vi "Basic Output demo.vi"() -> ()   [LabVIEW 2013]
panel:
  out "x .or. y?":bool
  in  "keyboard loop (ms)":u32=150
  in  "mouse loop (ms)":u32=100
  in  "keyboard service name":string="keyboard"
  in  "mouse service name":string="mouse"
  in  "Server address":string
  in  "trig left down":bool
  in  "trig left up":bool=TRUE
  in  "mode":T1(ring)
  out "Mouse Co-ords":T2
  in  "stop":bool
  out "Output (VKeys)":u8[](array[ring])
  # "Paste server address here!"
  # "SERVER DETAILS"
  # "TCP IP FOR KEYBOARD"
  # "&"
  # "DATASOCKET DETAILS  FOR MOUSE"
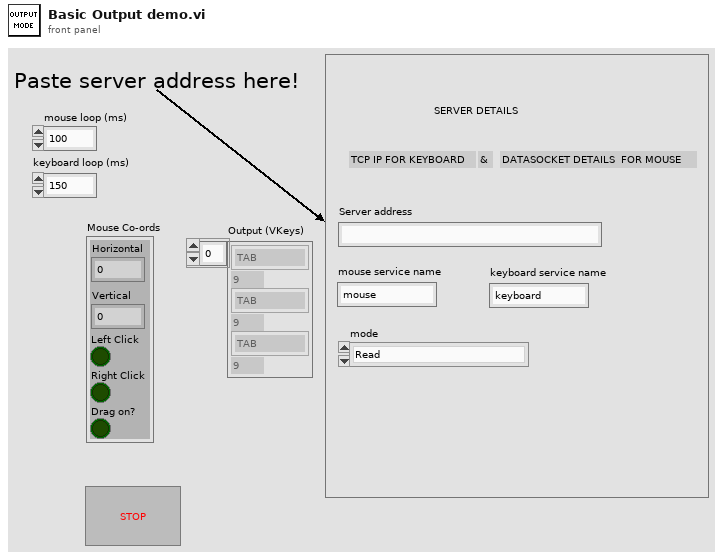
[diagram p1: front panel]
types:
  T1 = enum16{"Read", "Write", "ReadWrite", "BufferedRead", "BufferedReadWrite"}
  T2 = cluster{"Horizontal":i32, "Vertical":i32, "Left Click":bool, "Right Click":bool, "Drag on?":bool}
  T3 = enum16{"0", "1", "2", "3", "4", "5", "6", "7", "8", "9", "A", "B", "C", "D", "E", "F", "G", "H", "I", "J", "K", "L", "M", "N", "O", "P", "Q", "R", "S", "T", "U", "V", "W", "X", "Y", "Z", "F1", "F2", "F3", "F4", "F5", "F6", "F7", "F8", "F9", "F10", "F11", "F12", "F13", "F14", "F15", "ADD", "BACK", "BACKSLASH", "CAPITAL", "COMMA", "DECIMAL", "DELETE", "DIVIDE", "DOWN", "END", "EQUALS", "ESCAPE", "GRAVE (`)", "HOME", "INSERT", "LBRACKET", "LCONTROL", "LEFT", "L ALT", "LSHIFT", "LWIN", "MINUS", "MULTIPLY", "NEXT", "NUMLOCK", "NUMPAD_0", "NUMPAD_1", "NUMPAD_2", "NUMPAD_3", "NUMPAD_4", "NUMPAD_5", "NUMPAD_6", "NUMPAD_7", "NUMPAD_8", "NUMPAD_9", "PAUSE", "PERIOD", "PRIOR (PG UP)", "RBRACKET", "RCONTROL", "RETURN", "RIGHT", "R ALT", "RSHIFT", "RWIN", "SCROLL", "SEMICOLON", "SLASH", "SPACE", "SUBTRACT", "TAB", "UP", "ENTER (num pad)", "' (quote)"}[]
  T4 = cluster{" Key":u8, "Action":enum16{"Press", "Up", "Down"}, "Delay (ms)":u32}
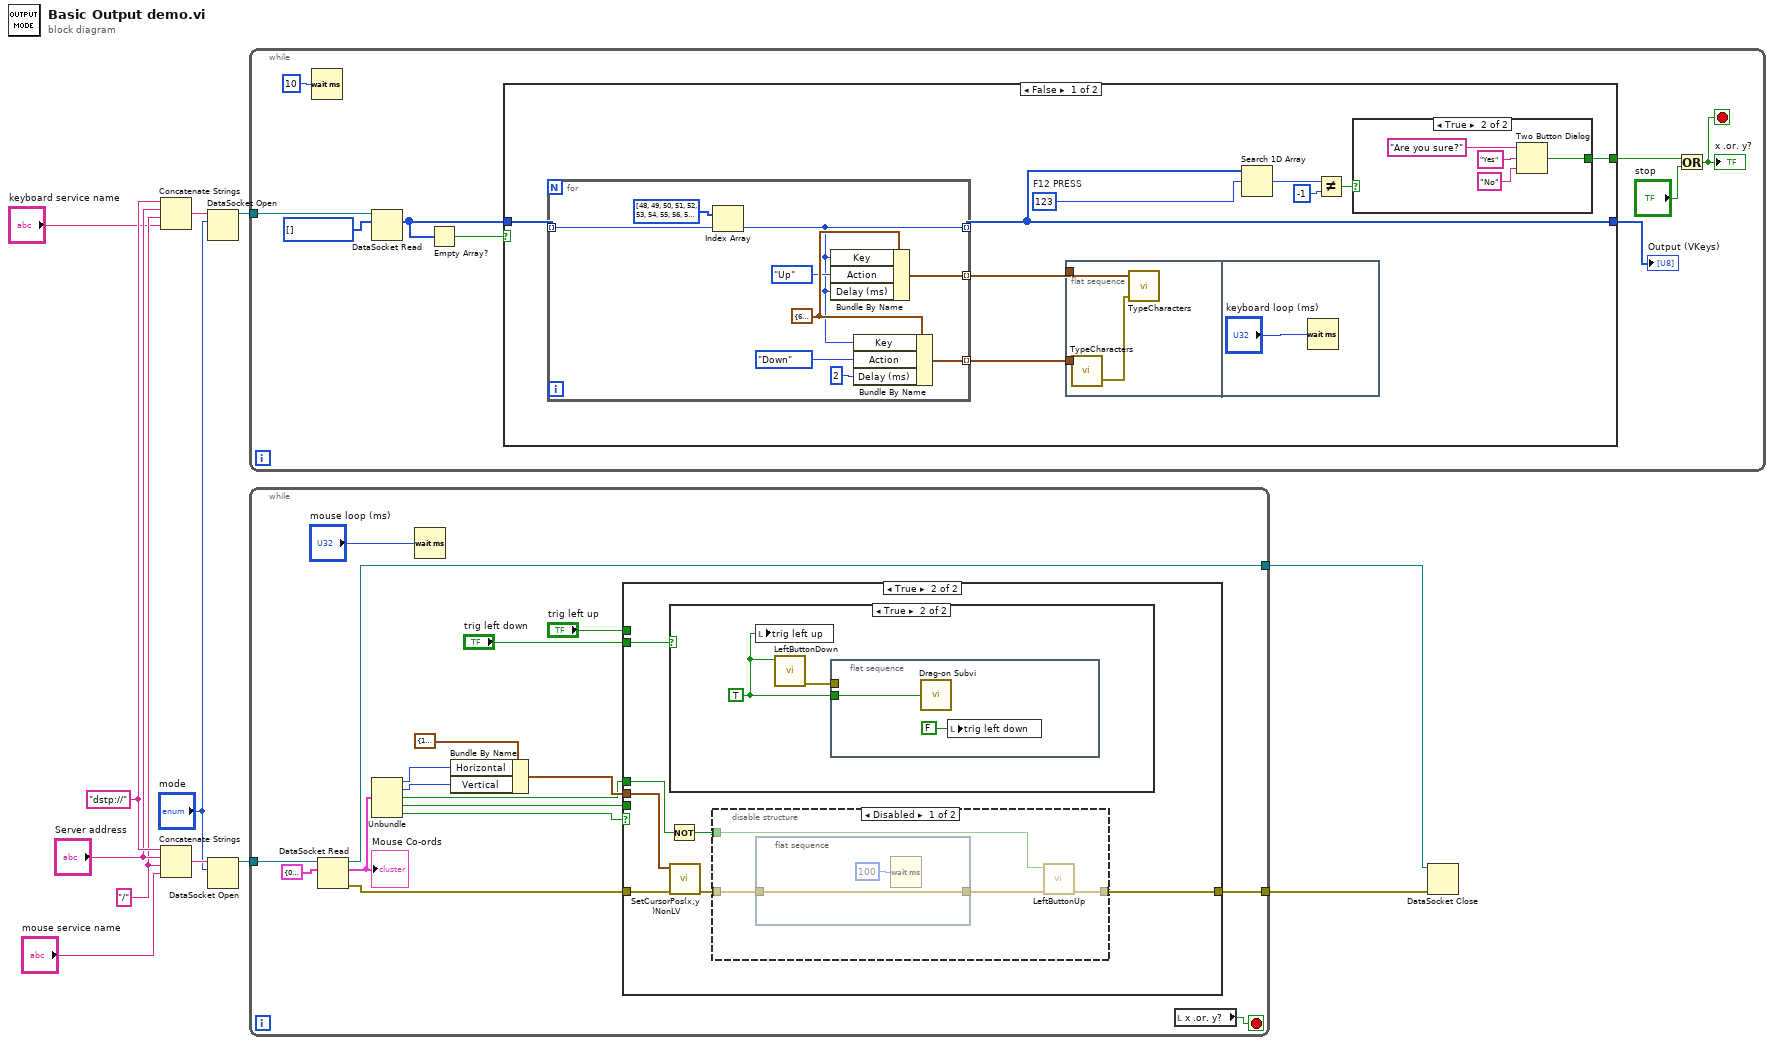
[diagram p0: block diagram]
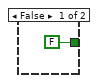
[diagram p2: hidden frame]
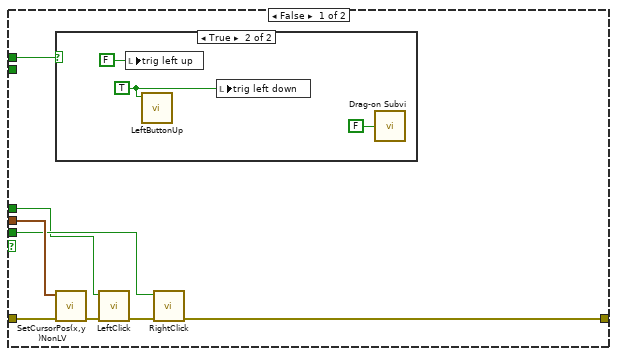
[diagram p4: hidden frame]
diagram:
  w5 = "/" ("string")
  w7 = "dstp://" ("string")
  n1 = Concatenate Strings(w7, "Server address", w5, "keyboard service name") -> (w3:string)
  n2 = Concatenate Strings(w7, "Server address", w5, "mouse service name") -> (w8:string)
  n3 = DataSocket Open(10:"mode", 11:w3) -> (3:w1:refnum<k13>)  [unwired: 2 in, 1 out]
  n4 = DataSocket Open(10:"mode", 11:w8) -> (3:w12:refnum<k13>)  [unwired: 2 in, 1 out]
  n5 = while {
    tunnel: w1 -> [w19]
    stop <- w20 stop-if-true
    w18 = T3 [] items=["0", "1", "2", "3", "4", "5", "6", "7", "8", "9", "A", "B", "C", "D", "E", "F", "G", "H", "I", "J", "K", "L", "M", "N", "O", "P", "Q", "R", "S", "T", "U", "V", "W", "X", "Y", "Z", "F1", "F2", "F3", "F4", "F5", "F6", "F7", "F8", "F9", "F10", "F11", "F12", "F13", "F14", "F15", "ADD", "BACK", "BACKSLASH", "CAPITAL", "COMMA", "DECIMAL", "DELETE", "DIVIDE", "DOWN", "END", "EQUALS", "ESCAPE", "GRAVE (`)", "HOME", "INSERT", "LBRACKET", "LCONTROL", "LEFT", "L ALT", "LSHIFT", "LWIN", "MINUS", "MULTIPLY", "NEXT", "NUMLOCK", "NUMPAD_0", "NUMPAD_1", "NUMPAD_2", "NUMPAD_3", "NUMPAD_4", "NUMPAD_5", "NUMPAD_6", "NUMPAD_7", "NUMPAD_8", "NUMPAD_9", "PAUSE", "PERIOD", "PRIOR (PG UP)", "RBRACKET", "RCONTROL", "RETURN", "RIGHT", "R ALT", "RSHIFT", "RWIN", "SCROLL", "SEMICOLON", "SLASH", "SPACE", "SUBTRACT", "TAB", "UP", "ENTER (num pad)", "' (quote)"] ("keys pressed")
    n6 = Wait (ms)(milliseconds to wait=u32 10) -> ()  [unwired: 1 out]
    n7 = DataSocket Read(10:w18, 11:w19) -> (2:w16:T3)  [unwired: 3 in, 6 out]
    n8 = Empty Array?(array=w16) -> (empty?=w15:bool)
    n9 = case shown="False" w15 {
      tunnel: w16 -> [w26 w49]
      tunnel: [w24 _] -> w17
      tunnel: [w22 w49] -> w13
      frame False {
        w27 = 123  # F12 PRESS
        n10 = for {
          tunnel: [w45] -> w30 mode=indexing
          tunnel: [w41] -> w22 mode=indexing
          tunnel: w26 -> [w44] mode=indexing
          tunnel: [w40] -> w23 mode=indexing
          w43 = T4 {" Key"=65, "Action"=enum."Press", "Delay (ms)"=10} ("Cluster")
          n11 = Index Array(array=i32[] [48, 49, 50, 51, 52, 53, 54, 55, 56, 57, 65, 66, 67, 68, 69, 70, 71, 72, 73, 74, 75, 76, 77, 78, 79, 80, 81, 82, 83, 84, 85, 86, 87, 88, 89, 90, 112, 113, 114, 115, 116, 117, 118, 119, 120, 121, 122, 123, 124, 125, 126, 107, 8, 220, 20, 188, 110, 46, 111, 40, 35, 187, 27, 192, 36, 45, 219, 162, 37, 18, 16, 91, 189, 106, 34, 144, 96, 97, 98, 99, 100, 101, 102, 103, 104, 105, 19, 190, 33, 221, 163, 13, 39, 165, 161, 92, 145, 186, 191, 32, 109, 9, 38, 13, 222], index=w44) -> (element=w41:i32)
          n12 = Bundle By Name(cluster=w43, "Key"=w41, "Action"=enum16{"Press", "Up", "Down"}."Up", "Delay (ms)"=w41) -> (w40:T4)
          n13 = Bundle By Name(cluster=w43, "Key"=w41, "Action"=enum16{"Press", "Up", "Down"}."Down", "Delay (ms)"=u32 2) -> (w45:T4)
        }
        n14 = flat-sequence {
          tunnel: w30 -> [w33]
          tunnel: w23 -> [w32]
          frame #0 {
            n15 = call "TypeCharacters.vi"("Key Array"=w33) -> ("error out"=w31:errorcluster)  [unwired: 3 in]
            n16 = call "TypeCharacters.vi"("error in (no error) 2"=w31, "Key Array"=w32) -> ()  [unwired: 2 in, 1 out]
          }
          frame #1 {
            n17 = Wait (ms)(milliseconds to wait="keyboard loop (ms)") -> ()  [unwired: 1 out]
          }
        }
        n18 = Search 1D Array(1D array=w22, element=w27) -> (index of element=w29:i32)  [unwired: 1 in]
        n19 = Not Equal?(x=w29, y=-1) -> (x != y?=w25:bool)
        n20 = case shown="True" w25 {
          tunnel: [FALSE ("T button?") w36] -> w24
          frame False {
          }
          frame True {
            n21 = Two Button Dialog(message="Are you sure?", 1:"No" ("F button name (\"Cancel\")"), 2:"Yes" ("T button name (\"OK\")")) -> (T button?=w36:bool)
          }
        }
      }
      frame True {
      }
    }
    "Output (VKeys)" <- w13
    n22 = Or(x=w17, y="stop") -> (x .or. y?=w20:bool)
    "x .or. y?" <- w20
  }
  n23 = while {
    tunnel: w12 -> [w66]
    tunnel: [w65] -> w11
    tunnel: [w54] -> w10
    stop <- w50 stop-if-true
    n24 = DataSocket Read(10:cluster{i32, i32, bool, bool, bool} {0, 0, TRUE, TRUE, TRUE}, 11:w66) -> (0:w55:errorcluster, 2:w63:cluster{i32, i32, bool, bool, bool}, 3:w65:refnum<k13>)  [unwired: 3 in, 4 out]
    "Mouse Co-ords" <- w63
    n25 = Unbundle(w63) -> (w60:i32, w59:i32, w56:bool, w58:bool, w52:bool)
    n26 = Wait (ms)(milliseconds to wait="mouse loop (ms)") -> ()  [unwired: 1 out]
    n27 = Bundle By Name(cluster=cluster{"Horizontal":i32, "Vertical":i32} {"Horizontal"=100, "Vertical"=100} ("RelativePosition"), "Horizontal"=w60, "Vertical"=w59) -> (w57:cluster{"Horizontal":i32, "Vertical":i32})
    n28 = case shown="True" w52 {
      tunnel: w57 -> [w74 w84]
      tunnel: w56 -> [w72 w83]
      tunnel: w58 -> [w73 _]
      tunnel: w55 -> [w67 w79]
      tunnel: [w70 w81] -> w54
      tunnel: "trig left up" -> [w68 _]
      tunnel: "trig left down" -> [_ w78]
      frame False {
        n29 = case shown="True" w68 {
          frame False {
          }
          frame True {
            w76 = TRUE ("Click?")
            n30 = local write "trig left up"(FALSE ("trig left up")) -> ()
            n31 = call "LeftButtonUp.vi"("Click?"=w76) -> ()  [unwired: 10 in, 1 out]
            n32 = local write "trig left down"(w76) -> ()
            n33 = call "Drag-on Subvi.vi"(FALSE) -> ()
          }
        }
        n34 = call "SetCursorPos(x,y)NonLV.vi"("error in"=w67, "RelativePosition"=w74) -> ("error out"=w69:errorcluster)  [unwired: 8 in, 1 out]
        n35 = call "LeftClick.vi"("Error in (no error)"=w69, "Click?"=w72) -> ("Error out"=w71:errorcluster)  [unwired: 9 in]
        n36 = call "RightClick.vi"("Error in (no error)"=w71, "Click?"=w73) -> ("Error out"=w70:errorcluster)  [unwired: 9 in]
      }
      frame True {
        n37 = Not(x=w83) -> (.not. x?=w82:bool)
        n38 = case shown="True" w78 {
          frame False {
          }
          frame True {
            w85 = TRUE ("Click?")
            n39 = local write "trig left up"(w85) -> ()
            n40 = call "LeftButtonDown.vi"("Click?"=w85) -> ("Error out"=w86:errorcluster)  [unwired: 10 in]
            n41 = flat-sequence {
              tunnel: w86 -> [_]
              tunnel: w85 -> [w87]
              frame #0 {
                n42 = call "Drag-on Subvi.vi"(w87) -> ()
                n43 = local write "trig left down"(FALSE ("trig left down")) -> ()
              }
            }
          }
        }
        n44 = call "SetCursorPos(x,y)NonLV.vi"("error in"=w79, "RelativePosition"=w84) -> ("error out"=w80:errorcluster)  [unwired: 8 in, 1 out]
        n45 = disable-structure shown="Disabled" {
          disable-tunnel: w82 -> [w91 _]
          disable-tunnel: w80 -> [w90 _]
          disable-tunnel: [w89 _] -> w81
          frame Disabled {
            n46 = flat-sequence {
              tunnel: w90 -> [w94]
              tunnel: [w94] -> w92
              frame #0 {
                n47 = Wait (ms)(milliseconds to wait=u32 100) -> ()  [unwired: 1 out]
              }
            }
            n48 = call "LeftButtonUp.vi"("Error in (no error)"=w92, "Click?"=w91) -> ("Error out"=w89:errorcluster)  [unwired: 9 in]
          }
          frame Enabled {
          }
        }
      }
    }
    n49 = local read "x .or. y?"() -> (w50:bool)
  }
  n50 = DataSocket Close(8:w10, 11:w11) -> ()  [unwired: 1 in, 2 out]
